vi "Climbing Sequence.vi"(10 "Stop":bool, 11 "Start Climb":bool) -> (1 "Winch Motor":dbl, 2 "Release claw":bool, 3 "Extension Solenoid":bool)   [LabVIEW 2015]
uses:
  Climbing claw.ctl
panel:
  in  "Climbing Time":dbl=10.0
  in  "Arm Forward Release":dbl=0.5
  out "Release climb arm":bool
  in  "Extend>retract delay":dbl=0.75 format="%#_13g"
  in  "Relase hook>extend delay":dbl=0.2 format="%#_13g"
  # "Solenoid used to extend arm up"
  # "Solenoid used to relase claw"
  # "Start squence//only works once"
  # "Output for whatever the winch motor is"
  # "Edit these when testing"
  # "Emergency stop"
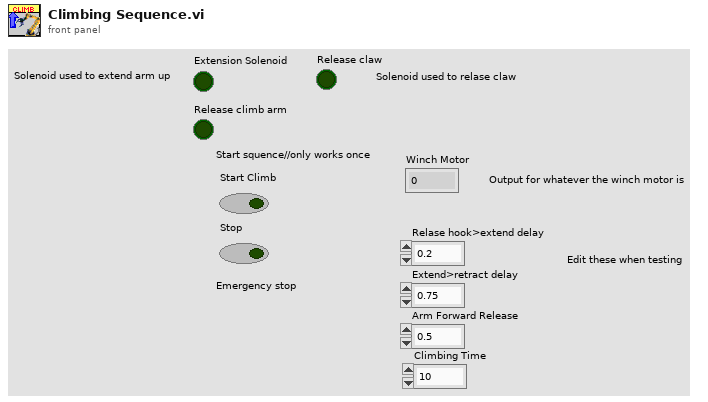
[diagram p1: front panel]
types:
  T1 = typedef "Climbing claw.ctl" = enum16{"Ready", "Extend", "Hook", "Retract", "Arm Forward", "Climb", "Stop"}
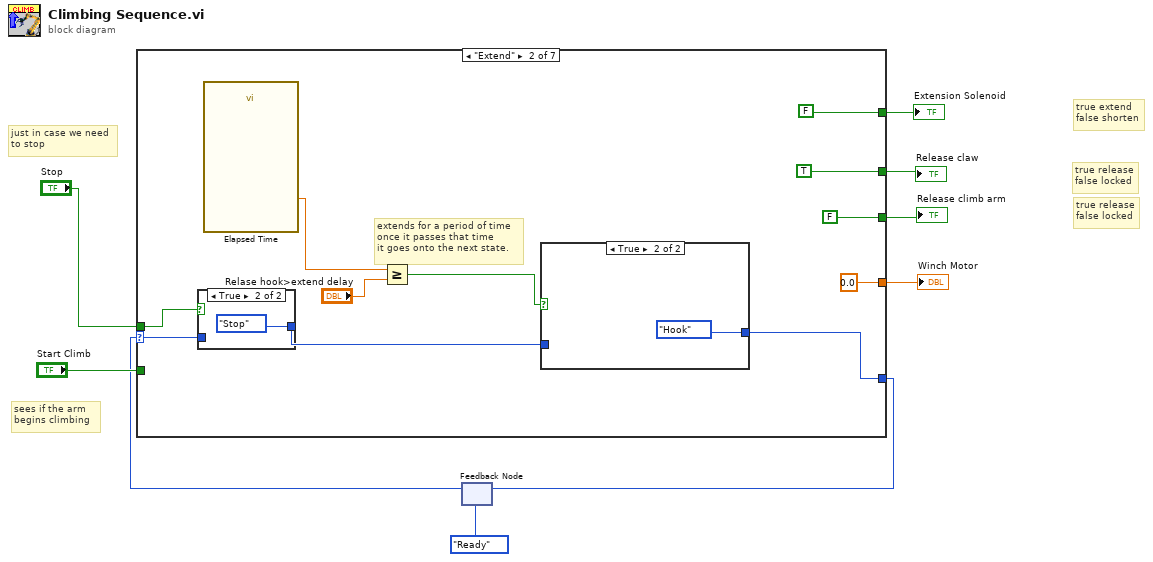
[diagram p0: block diagram]
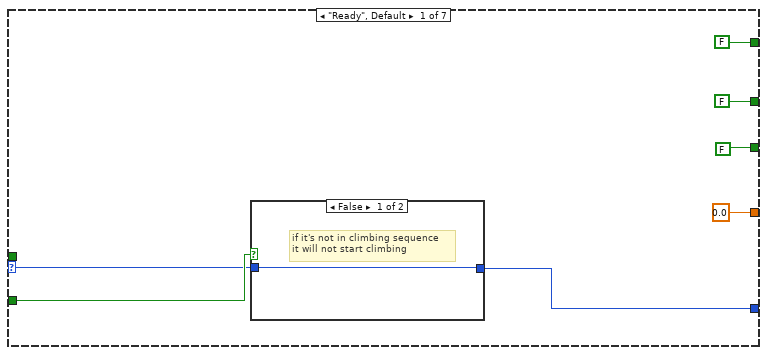
[diagram p2: hidden frame]
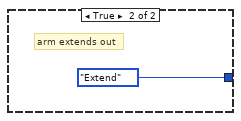
[diagram p3: hidden frame]
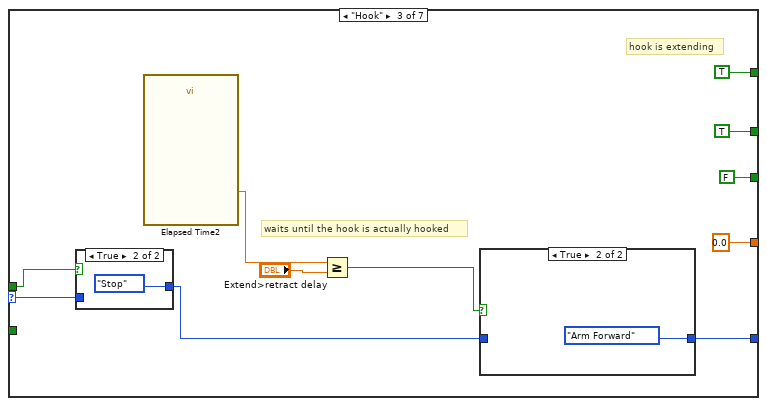
[diagram p6: hidden frame]
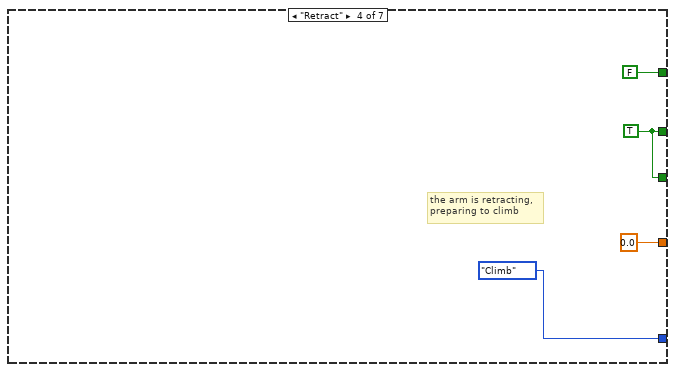
[diagram p9: hidden frame]
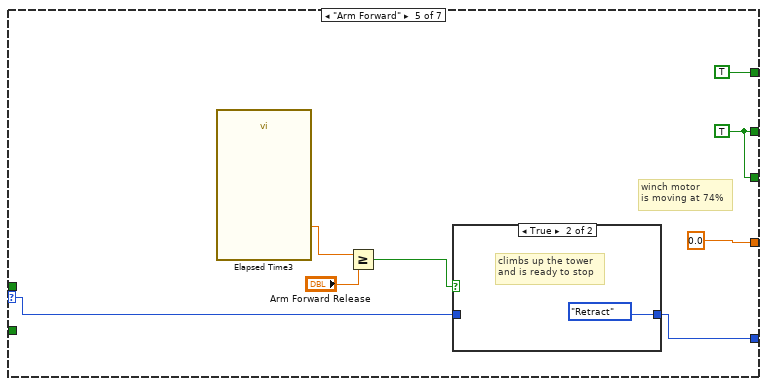
[diagram p10: hidden frame]
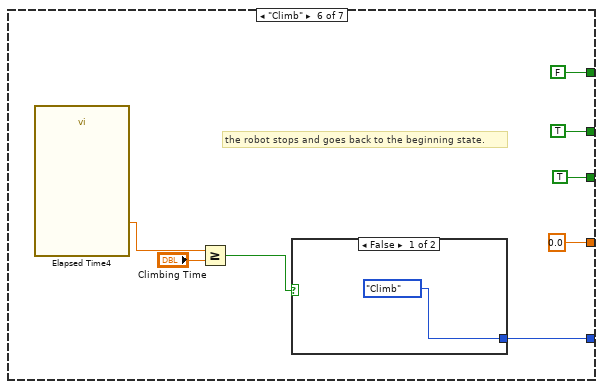
[diagram p12: hidden frame]
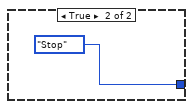
[diagram p13: hidden frame]
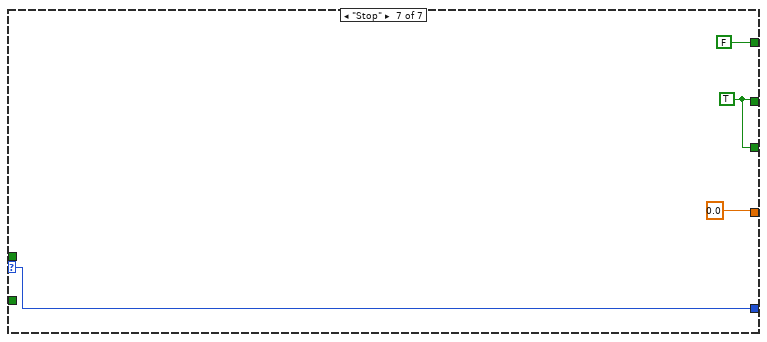
[diagram p14: hidden frame]
diagram:
  # "true release\nfalse locked"
  # "true release\nfalse locked"
  # "true extend\nfalse shorten"
  # "just in case we need\nto stop"
  # "sees if the arm\nbegins climbing"
  n1 = feedback #1(Climbing_claw."Ready") -> (w2:T1)
  n2 = case shown="\"Extend\"" w2 {
    selector: w2 -> [w11 w21 w38 _ w58 _ w73]
    tunnel: [w16 w29 w39 Climbing_claw."Climb" w59 w66 w73] -> w1
    tunnel: [FALSE FALSE TRUE FALSE TRUE FALSE FALSE] -> w9
    tunnel: [FALSE TRUE TRUE w49 w56 TRUE w75] -> w8
    tunnel: [0.0 0.0 0.0 0.0 0.0 0.0 0.0] -> w7
    tunnel: "Stop" -> [_ w22 w35 _ _ _ _]
    tunnel: "Start Climb" -> [w12 _ _ _ _ _ _]
    tunnel: [FALSE FALSE FALSE w49 w56 TRUE w75] -> w4
    frame "Ready", Default {
      n3 = case shown="False" w12 {
        tunnel: [w17 Climbing_claw."Extend"] -> w16
        tunnel: w11 -> [w17 _]
        frame False {
          # "if it's not in climbing sequence\nit will not start climbing"
        }
        frame True {
          # "arm extends out"
        }
      }
    }
    frame "Extend" {
      # "extends for a period of time\nonce it passes that time\nit goes onto the next state."
      n4 = case shown="True" w22 {
        tunnel: w21 -> [w30 _]
        tunnel: [w30 Climbing_claw."Stop"] -> w20
        frame False {
        }
        frame True {
        }
      }
      n5 = call "Elapsed Time"() -> ("Elapsed Time (s)"=w28:dbl)  [unwired: 12 in, 7 out]
      n6 = Greater Or Equal?(x=w28, y="Relase hook>extend delay") -> (x >= y?=w27:bool)
      n7 = case shown="True" w27 {
        tunnel: [w32 Climbing_claw."Hook"] -> w29
        tunnel: w20 -> [w32 _]
        frame False {
        }
        frame True {
        }
      }
    }
    frame "Hook" {
      # "waits until the hook is actually hooked"
      # "hook is extending"
      n8 = case shown="True" w35 {
        tunnel: [w45 Climbing_claw."Stop"] -> w37
        tunnel: w38 -> [w45 _]
        frame False {
        }
        frame True {
        }
      }
      n9 = call "Elapsed Time2"() -> ("Elapsed Time (s)"=w42:dbl)  [unwired: 12 in, 7 out]
      n10 = Greater Or Equal?(x=w42, y="Extend>retract delay") -> (x >= y?=w40:bool)
      n11 = case shown="True" w40 {
        tunnel: [w47 Climbing_claw."Arm Forward"] -> w39
        tunnel: w37 -> [w47 _]
        frame False {
        }
        frame True {
        }
      }
    }
    frame "Retract" {
      w49 = TRUE
      # "the arm is retracting, \npreparing to climb"
    }
    frame "Arm Forward" {
      w56 = TRUE
      # "winch motor\nis moving at 74%"
      n12 = call "Elapsed Time3"() -> ("Elapsed Time (s)"=w55:dbl)  [unwired: 12 in, 7 out]
      n13 = Greater Or Equal?(x=w55, y="Arm Forward Release") -> (x >= y?=w53:bool)
      n14 = case shown="True" w53 {
        tunnel: [w61 Climbing_claw."Retract"] -> w59
        tunnel: w58 -> [w61 _]
        frame False {
          # "it does not climb if it's false\nit does nothing"
        }
        frame True {
          # "climbs up the tower\nand is ready to stop"
        }
      }
    }
    frame "Climb" {
      # "the robot stops and goes back to the beginning state."
      n15 = call "Elapsed Time4"() -> ("Elapsed Time (s)"=w65:dbl)  [unwired: 12 in, 7 out]
      n16 = Greater Or Equal?(x=w65, y="Climbing Time") -> (x >= y?=w63:bool)
      n17 = case shown="False" w63 {
        tunnel: [Climbing_claw."Climb" Climbing_claw."Stop"] -> w66
        frame False {
        }
        frame True {
        }
      }
    }
    frame "Stop" {
      w75 = TRUE
    }
  }
  "Extension Solenoid" <- w9
  "Release claw" <- w8
  "Winch Motor" <- w7
  "Release climb arm" <- w4
  n18 = feedback-in #1(w1) -> ()
